vi "On Panel Close.vi"(8 "error in (no error)":errorcluster, 11 "App in":refnum<class "App.lvclass">) -> (0 "error out":errorcluster, 3 "App out":refnum<class "App.lvclass">)   [LabVIEW 2020, in "AR Example.lvlib" / "App.lvclass"]
uses:
  App.lvclass
  App.lvclass/App.ctl
  UI/UI.lvclass
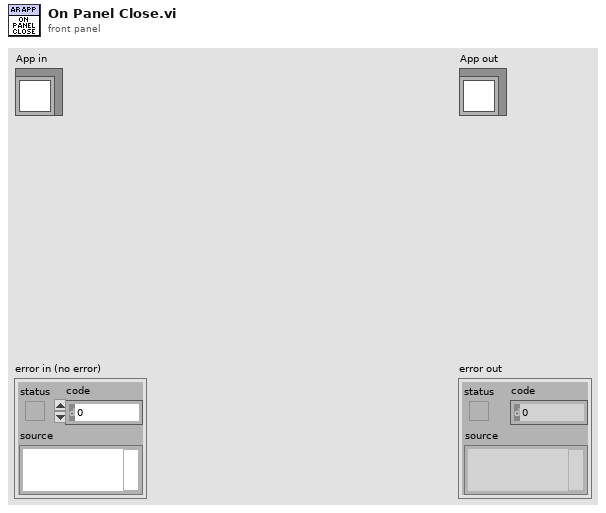
[diagram p1: front panel]
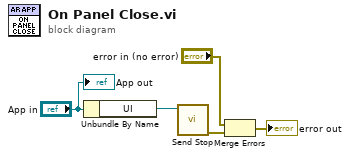
[diagram p0: block diagram]
diagram:
  n1 = Unbundle By Name("App in") -> ("UI"=w4:refnum<class "UI.lvclass">)
  n2 = call-dynamic "Send Stop.vi"("UI in"=w4) -> ("error out"=w3:errorcluster)  [unwired: 10 in]
  n3 = Merge Errors("error in (no error)", w3) -> (→"error out":errorcluster)
  "App out" <- "App in"
